vi "Get - Transfer Function.vi"(0 "reference in":refnum<class "GSwFormDSP.lvclass">, 5 "error in (no error)":errorcluster, 6 "Transfer Function Type":T1) -> (11 "Nb Averages":i32[](array[numeric]), 13 "Data":waveform(dbl)[](array[waveform]), 14 "reference out":refnum<class "GSwFormDSP.lvclass">, 19 "error out":errorcluster)   [LabVIEW 2022 SP3, in "GSwFormDSP.lvclass"]
uses:
  GSwFormDSP.lvclass
  functions/Transfer Function Type.ctl
  <vilib>/Analysis/NI_AALPro.lvlib
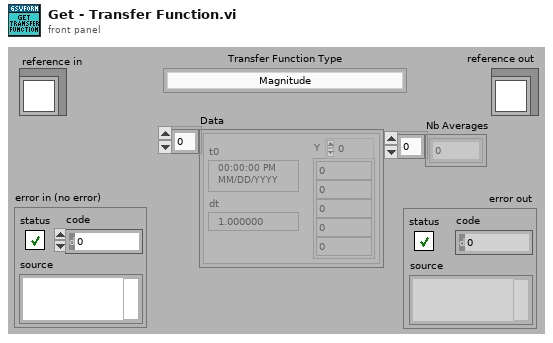
[diagram p1: front panel]
types:
  T1 = typedef "GSwFormDSP.lvclass/Transfer Function Type.ctl" = enum16{"Magnitude", "Phase (Rad)", "Phase Unwrap (Rad)", "Phase (Degree)", "Phase Unwrap (Degree)", "Coherence"}
  T2 = typedef "GSwFormDSP.lvclass/ObjectAttributes.ctl" = cluster{"Wform Ref":refnum<data-value>, "Nb Signals":i32, "Spectral Function Parameters":T3, "FFT":waveform(cdb)[], "Nb FFT":i32, "Nb Averages":i32[], "Reference Indexes":i32[], "Response Indexes":i32[], "Coherence":waveform(dbl)[], "TDF Parameters":T5, "DAQ":cluster{"Duration (sec)":dbl, "Buffer Size (Samples)":i32, "Offset (Samples)":i32}, "Filter Impulse Response (TDF)":waveform(dbl), "Sound Playback":T6}
  T3 = typedef "GSwFormDSP.lvclass/Spectral Parameters.ctl" = cluster{"Frequency resolution (Hz)":dbl, "Overlap":dbl, "Window":T4}
  T4 = typedef "NI_AALPro.lvlib/windowTd.ctl" = u32
  T5 = typedef "GSwFormDSP.lvclass/TDF Parameters.ctl" = cluster{"Filter":enum32{"Lowpass", "Highpass", "Bandpass", "Bandstop"}, "Type:":enum16{"Butterworth", "Chebyshev", "Inv Chebyshev", "Elliptic", "Bessel"}, "LP cutoff freq":dbl, "HP cutoff freq":dbl, "Order":i32, "passband ripple (dB)":dbl, "stopband attenuation (dB)":dbl, "Phaseless Filter":bool, "Include Fade IN and OUT":bool}
  T6 = typedef "GSwFormDSP.lvclass/Sound Playback.ctl" = cluster{"Timer start (ms)":u32, "task ID":T7, "Cursor Init Location (s)":dbl, "SC Volume":dbl}
  T7 = typedef "Sound Output Task ID.ctl" = u32
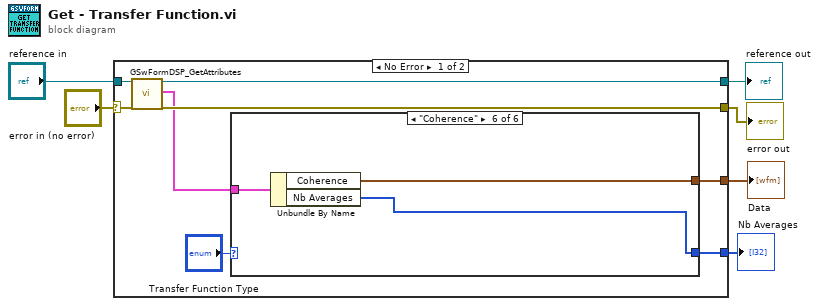
[diagram p0: block diagram]
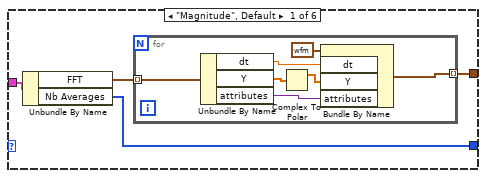
[diagram p2: hidden frame]
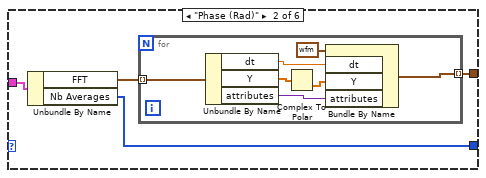
[diagram p3: hidden frame]
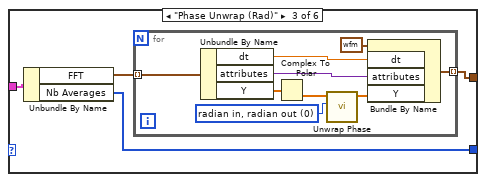
[diagram p4: hidden frame]
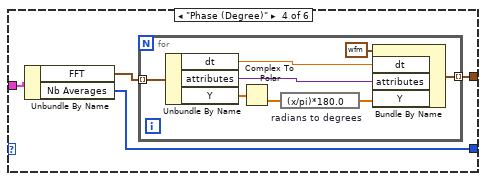
[diagram p5: hidden frame]
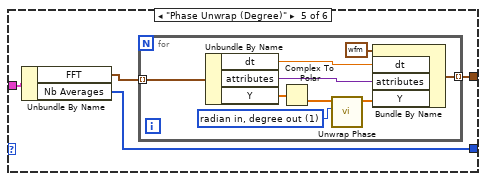
[diagram p6: hidden frame]
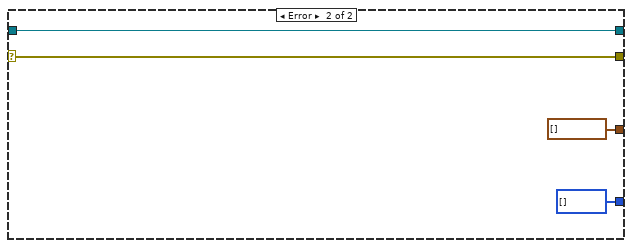
[diagram p7: hidden frame]
diagram:
  n1 = case shown="No Error" "error in (no error)" {
    selector: "error in (no error)" -> [w14 w81]
    tunnel: [w13 w81] -> w5
    tunnel: [w12 w80] -> w3
    tunnel: "reference in" -> [w11 w80]
    tunnel: [w9 waveform(dbl)[] [] ("Coherence")] -> w2
    tunnel: [w7 i32[] [] ("Nb Averages")] -> w1
    frame No Error {
      n2 = call "GSwFormDSP_GetAttributes.vi"("reference in"=w11, "error in (no error)"=w14) -> ("reference out"=w12:refnum<class "GSwFormDSP.lvclass">, "attributes"=w10:T2, "error out"=w13:errorcluster)  [unwired: 14 in, 1 out]
      n3 = case shown="\"Coherence\"" "Transfer Function Type" {
        tunnel: w10 -> [w18 w29 w40 w53 w65 w77]
        tunnel: [w15 w27 w37 w51 w62 w76] -> w9
        tunnel: [w17 w28 w39 w52 w64 w75] -> w7
        frame "Magnitude", Default {
          n4 = Unbundle By Name(w18) -> ("FFT"=w16:waveform(cdb)[], "Nb Averages"=w17:i32[])
          n5 = for {
            tunnel: w16 -> [w21] mode=indexing
            tunnel: [w20] -> w15 mode=indexing
            n6 = Unbundle By Name(w21) -> ("dt"=w23:dbl, "Y"=w25:cdb[], "attributes"=w22:variant)
            n7 = Complex To Polar(r * e^(i*theta)=w25) -> (r=w24:dbl[])  [unwired: 1 out]
            n8 = Bundle By Name(cluster=waveform(dbl) {"t0"=timestamp(0 s since 1904-01-01), "dt"=1.0, "Y"=[]} ("waveform"), "dt"=w23, "Y"=w24, "attributes"=w22) -> (w20:waveform(dbl))
          }
        }
        frame "Phase (Rad)" {
          n9 = Unbundle By Name(w29) -> ("FFT"=w26:waveform(cdb)[], "Nb Averages"=w28:i32[])
          n10 = for {
            tunnel: w26 -> [w33] mode=indexing
            tunnel: [w32] -> w27 mode=indexing
            n11 = Unbundle By Name(w33) -> ("dt"=w35:dbl, "Y"=w36:cdb[], "attributes"=w34:variant)
            n12 = Complex To Polar(r * e^(i*theta)=w36) -> (theta=w30:dbl[])  [unwired: 1 out]
            n13 = Bundle By Name(cluster=waveform(dbl) {"t0"=timestamp(0 s since 1904-01-01), "dt"=1.0, "Y"=[]} ("waveform"), "dt"=w35, "Y"=w30, "attributes"=w34) -> (w32:waveform(dbl))
          }
        }
        frame "Phase Unwrap (Rad)" {
          n14 = Unbundle By Name(w40) -> ("FFT"=w38:waveform(cdb)[], "Nb Averages"=w39:i32[])
          n15 = for {
            tunnel: w38 -> [w48] mode=indexing
            tunnel: [w47] -> w37 mode=indexing
            w43 = 0 items=["radian in, radian out", "radian in, degree out", "degree in, degree out", "degree in, radian out"] ("phase unit")
            n16 = Unbundle By Name(w48) -> ("dt"=w49:dbl, "attributes"=w45:variant, "Y"=w44:cdb[])
            n17 = Complex To Polar(r * e^(i*theta)=w44) -> (theta=w42:dbl[])  [unwired: 1 out]
            n18 = call <vilib>:"Unwrap Phase.vi"("phase unit"=w43, "Phase"=w42) -> ("Unwrapped Phase"=w41:dbl[])  [unwired: 8 in, 1 out]
            n19 = Bundle By Name(cluster=waveform(dbl) {"t0"=timestamp(0 s since 1904-01-01), "dt"=1.0, "Y"=[]} ("waveform"), "dt"=w49, "attributes"=w45, "Y"=w41) -> (w47:waveform(dbl))
          }
        }
        frame "Phase (Degree)" {
          n20 = Unbundle By Name(w53) -> ("FFT"=w50:waveform(cdb)[], "Nb Averages"=w52:i32[])
          n21 = for {
            tunnel: w50 -> [w60] mode=indexing
            tunnel: [w59] -> w51 mode=indexing
            n22 = Unbundle By Name(w60) -> ("dt"=w61:dbl, "attributes"=w57:variant, "Y"=w56:cdb[])
            n23 = Complex To Polar(r * e^(i*theta)=w56) -> (theta=w55:dbl[])  [unwired: 1 out]
            n24 = expression code="(x/pi)*180.0" "radians to degrees"(w55) -> (w54:dbl[])
            n25 = Bundle By Name(cluster=waveform(dbl) {"t0"=timestamp(0 s since 1904-01-01), "dt"=1.0, "Y"=[]} ("waveform"), "dt"=w61, "attributes"=w57, "Y"=w54) -> (w59:waveform(dbl))
          }
        }
        frame "Phase Unwrap (Degree)" {
          n26 = Unbundle By Name(w65) -> ("FFT"=w63:waveform(cdb)[], "Nb Averages"=w64:i32[])
          n27 = for {
            tunnel: w63 -> [w73] mode=indexing
            tunnel: [w72] -> w62 mode=indexing
            w68 = 1 items=["radian in, radian out", "radian in, degree out", "degree in, degree out", "degree in, radian out"] ("phase unit")
            n28 = Unbundle By Name(w73) -> ("dt"=w74:dbl, "attributes"=w70:variant, "Y"=w69:cdb[])
            n29 = Complex To Polar(r * e^(i*theta)=w69) -> (theta=w67:dbl[])  [unwired: 1 out]
            n30 = call <vilib>:"Unwrap Phase.vi"("phase unit"=w68, "Phase"=w67) -> ("Unwrapped Phase"=w66:dbl[])  [unwired: 8 in, 1 out]
            n31 = Bundle By Name(cluster=waveform(dbl) {"t0"=timestamp(0 s since 1904-01-01), "dt"=1.0, "Y"=[]} ("waveform"), "dt"=w74, "attributes"=w70, "Y"=w66) -> (w72:waveform(dbl))
          }
        }
        frame "Coherence" {
          n32 = Unbundle By Name(w77) -> ("Coherence"=w76:waveform(dbl)[], "Nb Averages"=w75:i32[])
        }
      }
    }
    frame Error {
    }
  }
  "error out" <- w5
  "reference out" <- w3
  "Data" <- w2
  "Nb Averages" <- w1
